vi "Update State.vi"(8 "error in (no error)":errorcluster, 11 "Alarm Handler Actor in":refnum<class "Alarm Handler Actor.lvclass">) -> (0 "error out":errorcluster, 3 "Alarm Handler Actor out":refnum<class "Alarm Handler Actor.lvclass">)   [LabVIEW 2015, in "Alarm Handler Actor.lvclass"]
uses:
  Alarm Handler Actor.lvclass
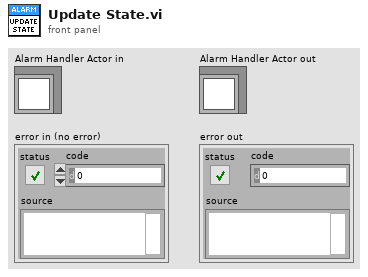
[diagram p1: front panel]
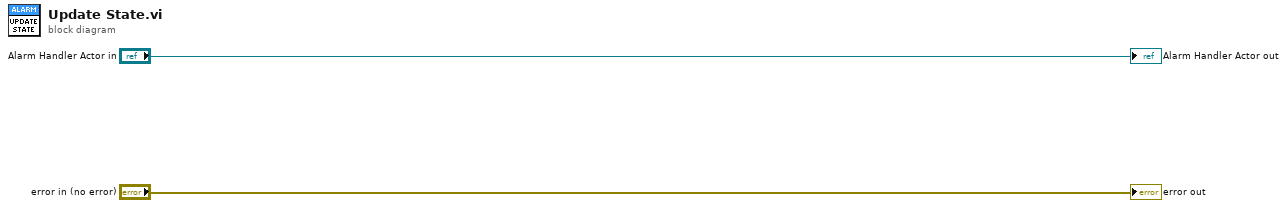
[diagram p0: block diagram]
diagram:
  "Alarm Handler Actor out" <- "Alarm Handler Actor in"
  "error out" <- "error in (no error)"
